vi "global python version.vi"() -> ()   [LabVIEW 2023]
panel:
  in  "Pyhton Version":string="3.12"
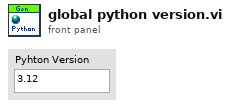
[diagram p1: front panel]
diagram:
